vi "userInputSetup.vi"(7 "Monochromator":T1={"Type"=enum."PTI", "Wavelength (nm)"=500.0, "Grating, gr/mm"=enum."1200", "Grating mode"=enum."IR", "Spectrum mode"={"Spectrum mode?"=FALSE, "Start wavelength (nm)"=0.0, "End wavelength (nm)"=0.0, "Wavelength step (nm)"=0.0, "Wavelength array"=[], "array index"=0}, "PTI"={"Delay before read (ms)"=1000, "Mono 1"={"Timeout (ms)"=1000, "Resource Name"="COM1", "Baud Rate"=9600, "Data Bits"=8, "Parity"=0, "Stop Bits"=10, "Flow Control"=0}, "Mono 2"={"Timeout (ms)"=1000, "Resource Name"="COM1", "Baud Rate"=9600, "Data Bits"=8, "Parity"=0, "Stop Bits"=10, "Flow Control"=0}, "Two PTI Monochromators?"=FALSE}, "Oriel (custom)"={"reference"=refnum}, "Force wavelength confirmation (PTI)?"=FALSE} {"PTI"."Mono 2"."Flow Control" items=["1.0"=10, "1.5"=15, "2.0"=20]; "PTI"."Mono 2"."Stop Bits" items=["None", "Odd", "Even", "Mark", "Space"]; "PTI"."Mono 2"."Parity" items=["None", "Odd", "Even", "Mark", "Space"]; "PTI"."Mono 1"."Flow Control" items=["1.0"=10, "1.5"=15, "2.0"=20]; "PTI"."Mono 1"."Stop Bits" items=["None", "Odd", "Even", "Mark", "Space"]; "PTI"."Mono 1"."Parity" items=["None", "Odd", "Even", "Mark", "Space"]}, 8 "error in (no error)":errorcluster, 10 "Wavelength (nm)":dbl, 11 "Enable wavelength input?":bool) -> (0 "error out":errorcluster, 5 "Monochromator out":T1={"Type"=enum."PTI", "Wavelength (nm)"=500.0, "Grating, gr/mm"=enum."1200", "Grating mode"=enum."Visible", "Spectrum mode"={"Spectrum mode?"=FALSE, "Start wavelength (nm)"=0.0, "End wavelength (nm)"=0.0, "Wavelength step (nm)"=0.0, "Wavelength array"=[], "array index"=0}, "PTI"={"Delay before read (ms)"=1000, "Mono 1"={"Timeout (ms)"=1000, "Resource Name"="COM1", "Baud Rate"=9600, "Data Bits"=8, "Parity"=0, "Stop Bits"=10, "Flow Control"=0}, "Mono 2"={"Timeout (ms)"=1000, "Resource Name"="COM1", "Baud Rate"=9600, "Data Bits"=8, "Parity"=0, "Stop Bits"=10, "Flow Control"=0}, "Two PTI Monochromators?"=FALSE}, "Oriel (custom)"={"reference"=refnum}, "Force wavelength confirmation (PTI)?"=FALSE} {"PTI"."Mono 2"."Flow Control" items=["1.0"=10, "1.5"=15, "2.0"=20]; "PTI"."Mono 2"."Stop Bits" items=["None", "Odd", "Even", "Mark", "Space"]; "PTI"."Mono 2"."Parity" items=["None", "Odd", "Even", "Mark", "Space"]; "PTI"."Mono 1"."Flow Control" items=["1.0"=10, "1.5"=15, "2.0"=20]; "PTI"."Mono 1"."Stop Bits" items=["None", "Odd", "Even", "Mark", "Space"]; "PTI"."Mono 1"."Parity" items=["None", "Odd", "Even", "Mark", "Space"]})   [LabVIEW 2017, in "Monochromator.lvlib" / "PTI.lvlib"]
uses:
  PTI.lvlib
  Controls/Grating.ctl
  Controls/Params.ctl
  Controls/Type.ctl
  Controls/GratingValues.ctl
  Controls/VISA parameters.ctl
  Custom Oriel drivers/Controls/Params.ctl
  C:/Project Work/icl-optical-software-rewrite/Optical Software Code Simplified/Modules/Monochromator/Cornerstone.dll
  Cornerstone.dll
  Monochromator.lvlib
  Serial comms/Serial comms.lvlib
  Custom Oriel drivers/Oriel (custom drivers).lvlib
panel:
  out "physical dial value":dbl format="(%#_g shown on dial)"
  in  "OK":bool caption="OK1"
  out "Please enter...":string
  out "Message":string
  in  "Grating":T4=enum."Visible"
  in  "Wavelength (nm)":u32=500 caption="Monochromator readout" max=1600 step=1
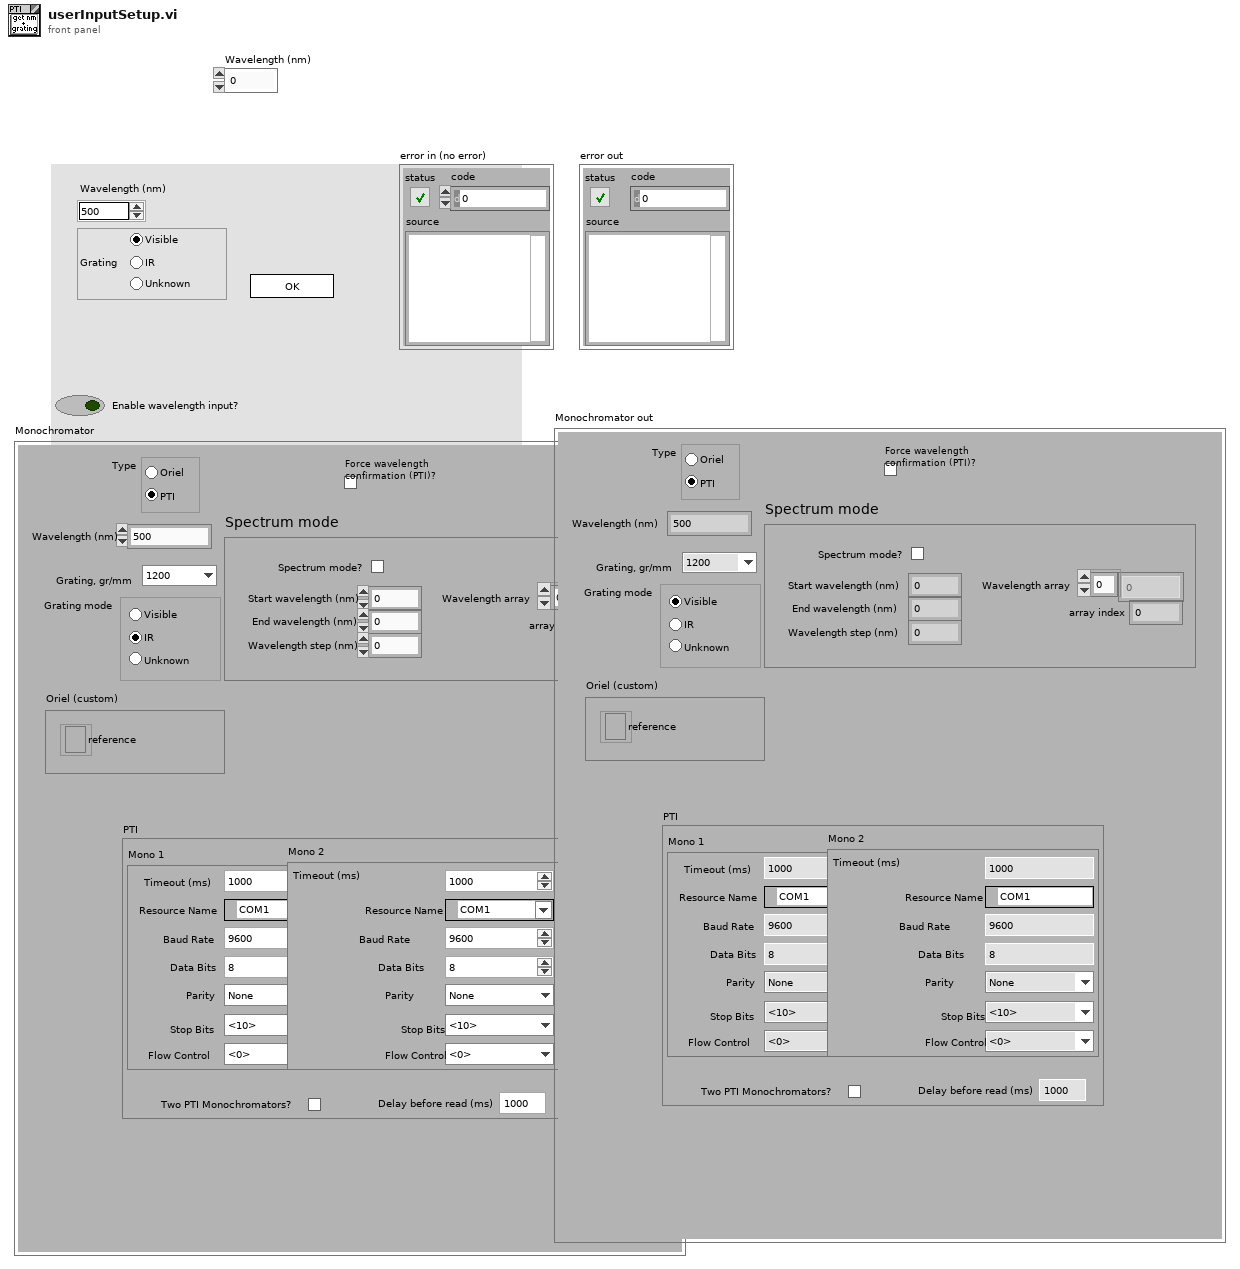
[diagram p1: front panel]
types:
  T1 = typedef "Monochromator.lvlib/Params.ctl" = cluster{"Type":T2, "Wavelength (nm)":dbl, "Grating, gr/mm":T3, "Grating mode":T4, "Spectrum mode":cluster{"Spectrum mode?":bool, "Start wavelength (nm)":dbl, "End wavelength (nm)":dbl, "Wavelength step (nm)":dbl, "Wavelength array":dbl[], "array index":u32}, "PTI":T5, "Oriel (custom)":T7, "Force wavelength confirmation (PTI)?":bool}
  T2 = typedef "Monochromator.lvlib/Type.ctl" = enum32{"Oriel", "PTI"}
  T3 = typedef "Monochromator.lvlib/GratingValues.ctl" = enum16{"2400", "1800", "1200", "600", "300", "150"}
  T4 = typedef "Monochromator.lvlib/Grating.ctl" = enum32{"Unknown", "Visible", "IR"}
  T5 = typedef "Monochromator.lvlib/PTI.lvlib/Params.ctl" = cluster{"Delay before read (ms)":u32, "Mono 1":T6, "Mono 2":T6, "Two PTI Monochromators?":bool}
  T6 = typedef "Serial comms.lvlib/VISA parameters.ctl" = cluster{"Timeout (ms)":u32, "Resource Name":refnum<visa-resource-name>, "Baud Rate":u32, "Data Bits":u16, "Parity":u16, "Stop Bits":u16, "Flow Control":u16}
  T7 = typedef "Monochromator.lvlib/Oriel (custom drivers).lvlib/Params.ctl" = cluster{"reference":refnum<k24>}
  T8 = enum8{"Enabled", "Disabled", "Disabled and Grayed Out"}
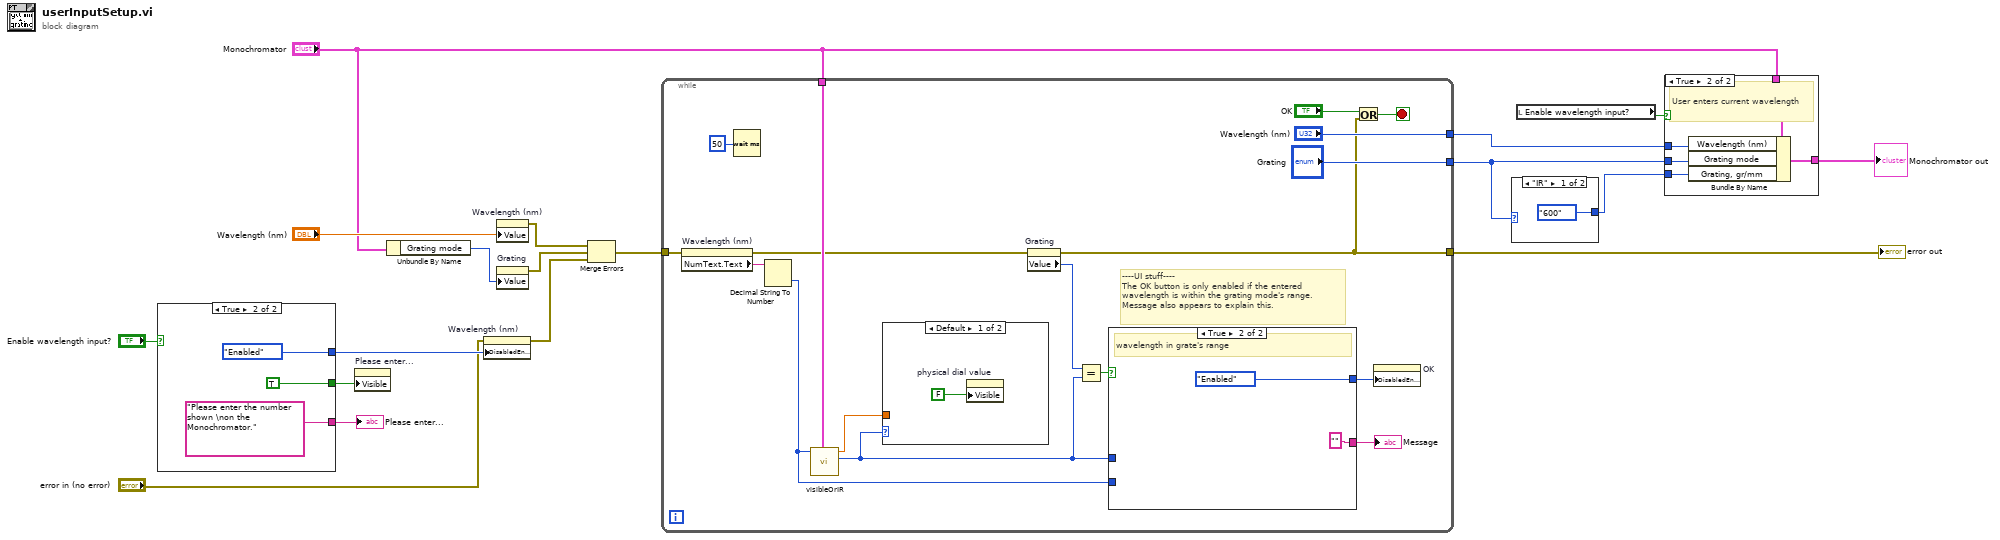
[diagram p0: block diagram]
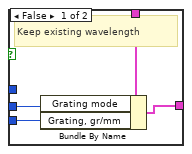
[diagram p2: hidden frame]
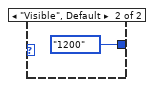
[diagram p3: hidden frame]
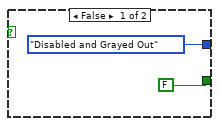
[diagram p4: hidden frame]
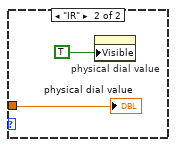
[diagram p5: hidden frame]
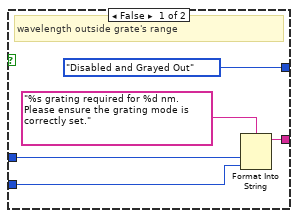
[diagram p6: hidden frame]
diagram:
  n1 = case shown="True" "Enable wavelength input?" {
    tunnel: [T8."Disabled and Grayed Out" ("Disabled") T8."Enabled" ("Disabled")] -> w12
    tunnel: [FALSE TRUE] -> w11
    tunnel: [_ "Please enter the number shown \non the Monochromator."] -> w1
    frame False {
    }
    frame True {
    }
  }
  "Please enter..." <- w1
  n2 = property on="Please enter..." class="Str"("Visible"=w11) -> ()  [unwired: 2 in, 2 out]
  n3 = Unbundle By Name("Monochromator") -> ("Grating mode"=w18:T4)
  n4 = property on="Wavelength (nm)" class="DigNum (strict)"(error in="error in (no error)", "DisabledEnum"=w12) -> (error out=w13:errorcluster)  [unwired: 1 in, 1 out]
  n5 = property on="Wavelength (nm)" class="DigNum (strict)"("Value"="Wavelength (nm)") -> (error out=w17:errorcluster)  [unwired: 2 in, 1 out]
  n6 = property on="Grating" class="RadioBtnsControl (strict)"("Value"=w18) -> (error out=w16:errorcluster)  [unwired: 2 in, 1 out]
  n7 = Merge Errors(w17, w16, w13) -> (w15:errorcluster)
  n8 = while {
    tunnel: "Monochromator" -> [w32]
    tunnel: ["Wavelength (nm)"] -> w8
    tunnel: ["Grating"] -> w7
    tunnel: w15 -> [w31]
    tunnel: [w26] -> w14
    stop <- w28 stop-if-true
    # "----UI stuff----\nThe OK button is only enabled if the entered wavelength is within the grating mode's range. Message also appears to explain this."
    n9 = property on="Wavelength (nm)" class="DigNum (strict)"(error in=w31) -> (error out=w30:errorcluster, "NumText.Text"=w39:string)  [unwired: 1 in, 1 out]
    n10 = Wait (ms)(milliseconds to wait=u32 50) -> ()  [unwired: 1 out]
    n11 = Decimal String To Number(string=w39) -> (number=w35:i32)  [unwired: 2 in, 1 out]
    n12 = call "visibleOrIR.vi"("Monochromator"=w32, "Wavelength (nm)"=w35) -> ("IR/visible"=w24:T4, "Displayed mono wavelength (nm)"=w25:dbl)  [unwired: 7 in, 1 out]
    n13 = case shown="Default" w24 {
      tunnel: w25 -> [_ w42]
      frame Default {
        n14 = property on="physical dial value" class="DigNum (strict)"("Visible"=FALSE) -> ()  [unwired: 2 in, 2 out]
      }
      frame "IR" {
        n15 = property on="physical dial value" class="DigNum (strict)"("Visible"=TRUE) -> ()  [unwired: 2 in, 2 out]
        "physical dial value" <- w42
      }
    }
    n16 = property on="Grating" class="RadioBtnsControl (strict)"(error in=w30) -> (error out=w26:errorcluster, "Value"=w34:T4)  [unwired: 1 in, 1 out]
    n17 = Equal?(x=w34, y=w24) -> (x = y?=w38:bool)
    n18 = case shown="True" w38 {
      tunnel: [T8."Disabled and Grayed Out" ("Disabled") T8."Enabled" ("Disabled")] -> w37
      tunnel: w24 -> [w45 _]
      tunnel: [w46 ""] -> w36
      tunnel: w35 -> [w44 _]
      frame False {
        # "wavelength outside grate's range"
        n19 = Format Into String(format string="%s grating required for %d nm. Please ensure the grating mode is correctly set.", w45, w44) -> (resulting string=w46:string)  [unwired: 2 in, 1 out]
      }
      frame True {
        # "wavelength in grate's range"
      }
    }
    "Message" <- w36
    n20 = Or(x="OK", y=w26) -> (x .or. y?=w28:bool)
    n21 = property on="OK" class="Bool"("DisabledEnum"=w37) -> ()  [unwired: 2 in, 2 out]
  }
  "error out" <- w14
  n22 = case shown="\"IR\"" w7 {
    tunnel: [GratingValues."600" ("Grating, gr/mm") GratingValues."1200" ("Grating, gr/mm")] -> w6
    frame "IR" {
    }
    frame "Visible", Default {
    }
  }
  n23 = local read "Enable wavelength input?"() -> (w9:bool)
  n24 = case shown="True" w9 {
    tunnel: "Monochromator" -> [w56 w61]
    tunnel: [w55 w60] -> w5
    tunnel: w8 -> [_ w59]
    tunnel: w7 -> [w54 w58]
    tunnel: w6 -> [w53 w57]
    frame False {
      # "Keep existing wavelength"
      n25 = Bundle By Name(cluster=w56, "Grating mode"=w54, "Grating, gr/mm"=w53) -> (w55:T1)
    }
    frame True {
      # "User enters current wavelength"
      n26 = Bundle By Name(cluster=w61, "Wavelength (nm)"=w59, "Grating mode"=w58, "Grating, gr/mm"=w57) -> (w60:T1)
    }
  }
  "Monochromator out" <- w5
